vi "about.vi"(7 "httpRequestID":u32) -> ()   [LabVIEW 2011]
doc: "This VI is a state machine that can be ran from a Browser."
uses:
  server/database/Users/User Record.ctl
  <vilib>/wsapi/NI_WebServices.lvlib
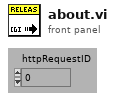
[diagram p1: front panel]
types:
  T1 = typedef "User Record.ctl" = cluster{"ixUser":i32, "sxUsername":string, "sLastName":string, "sFirstName":string, "sEmail":string, "sPassword":string, "tLoginTime":timestamp, "sLoginComputer":string, "fAdministrator":bool, "fRunSequences":bool, "fModifySequences":bool, "fRunScenarios":bool, "fModifyScenarios":bool, "fModifyTemplates":bool, "fModifyUsers":bool, "fModifyStations":bool, "fModifyFields":bool}
  T2 = typedef "Connection Refnum.ctl" = cluster{"Environment Handle":i32, "Connection Handle":i32}
  T3 = typedef "Keyed Array.ctl" = cluster{"keys":string[], "values":string[]}
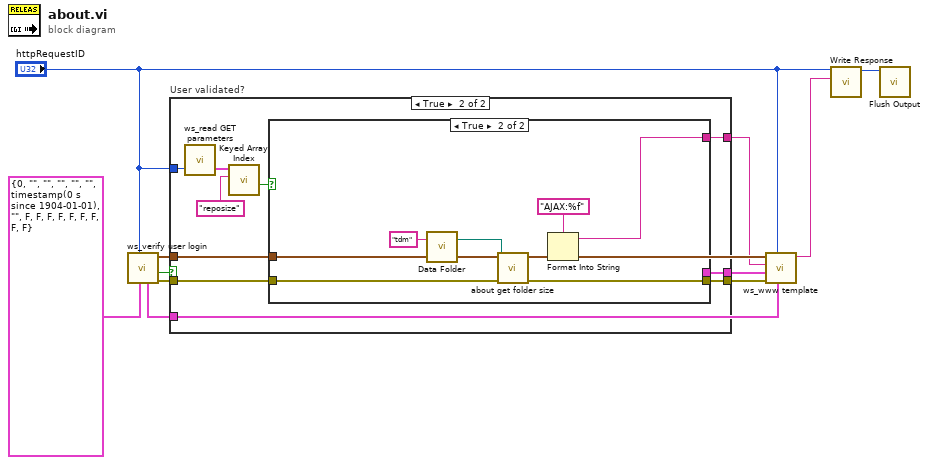
[diagram p0: block diagram]
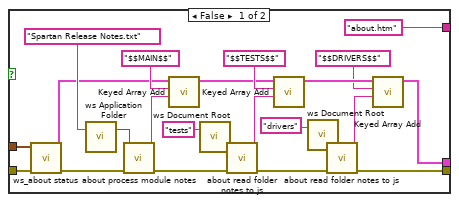
[diagram p3: hidden frame]
diagram:
  n1 = call "ws_verify user login.vi"("Required Permisions"=T1 {"ixUser"=0, "sxUsername"="", "sLastName"="", "sFirstName"="", "sEmail"="", "sPassword"="", "tLoginTime"=timestamp(0 s since 1904-01-01), "sLoginComputer"="", "fAdministrator"=FALSE, "fRunSequences"=FALSE, "fModifySequences"=FALSE, "fRunScenarios"=FALSE, "fModifyScenarios"=FALSE, "fModifyTemplates"=FALSE, "fModifyUsers"=FALSE, "fModifyStations"=FALSE, "fModifyFields"=FALSE} ("User Record"), "httpRequestID"="httpRequestID") -> ("error out"=w9:errorcluster, "User Verified\nand Spartan\nAuthorized?"=w11:bool, "DB Connection Ref"=w6:T2, "User"=w3:T1)  [unwired: 6 in]
  n2 = case "User validated?" shown="True" w11 {
    tunnel: [w12 w18] -> w7
    tunnel: [_ w21] -> w4
    tunnel: [_ w20] -> w5
    tunnel: w3 -> [_ _]
    tunnel: w9 -> [w12 w19]
    tunnel: w6 -> [_ w17]
    tunnel: "httpRequestID" -> [_ w16]
    frame False {
    }
    frame True {
      n3 = call "ws_read GET parameters.vi"("httpRequestID"=w16) -> ("GET query params"=w15:T3)  [unwired: 2 in]
      n4 = call <vilib>:"Keyed Array Index.vi"("key"="reposize", "array in"=w15) -> ("valid key"=w14:bool)  [unwired: 2 in, 3 out]
      n5 = case shown="True" w14 {
        tunnel: ["about.htm" ("Template (\"\")") w50] -> w21
        tunnel: [w41 _] -> w20
        tunnel: w19 -> [w32 w49]
        tunnel: [w31 w45] -> w18
        tunnel: w17 -> [w28 _]
        frame False {
          n6 = call "ws_about status.vi"("error in (no error)"=w32, "Connection Refnum"=w28) -> ("error out"=w35:errorcluster, "keys"=w25:T3)  [unwired: 8 in]
          n7 = call "ws Application Folder.vi"("Relative Path (\"\" - Folder)"="Spartan Release Notes.txt" ("name or relative path")) -> ("Application Folder"=w33:path)  [unwired: 2 in]
          n8 = call "about process module notes.vi"("error in (no error)"=w35, "Notes Path (empty)"=w33) -> ("error out"=w34:errorcluster, "release notes obj"=w29:string)  [unwired: 8 out]
          n9 = call <vilib>:"Keyed Array Add.vi"("value"=w29, "key"="$$MAIN$$" ("Template (\"\")"), "array in"=w25) -> ("array out"=w39:T3)  [unwired: 2 in, 2 out]
          n10 = call "ws Document Root.vi"("Relative Path (\"\" - Folder)"="tests" ("Template (\"\")")) -> ("DocumentRoot Folder"=w37:path)  [unwired: 2 in]
          n11 = call "about read folder notes to js.vi"("error in (no error)"=w34, "Modules Path (empty)"=w37) -> ("error out"=w36:errorcluster, "Module Notes objects"=w27:string)  [unwired: 8 out]
          n12 = call <vilib>:"Keyed Array Add.vi"("value"=w27, "key"="$$TESTS$$" ("Template (\"\")"), "array in"=w39) -> ("array out"=w42:T3)  [unwired: 2 in, 2 out]
          n13 = call "ws Document Root.vi"("Relative Path (\"\" - Folder)"="drivers" ("Template (\"\")")) -> ("DocumentRoot Folder"=w23:path)  [unwired: 2 in]
          n14 = call "about read folder notes to js.vi"("error in (no error)"=w36, "Modules Path (empty)"=w23) -> ("error out"=w31:errorcluster, "Module Notes objects"=w26:string)  [unwired: 8 out]
          n15 = call <vilib>:"Keyed Array Add.vi"("value"=w26, "key"="$$DRIVERS$$" ("Template (\"\")"), "array in"=w42) -> ("array out"=w41:T3)  [unwired: 2 in, 2 out]
        }
        frame True {
          n16 = call "Data Folder.vi"("Relative Path (\"\" - Folder)"="tdm" ("Relative Path (\"\" - Folder)")) -> ("Data Folder"=w48:path)  [unwired: 2 in]
          n17 = call "about get folder size.vi"("error in (no error)"=w49, "Directory Path"=w48) -> ("error out"=w45:errorcluster, "Disk Space Used (MB)"=w46:dbl)  [unwired: 8 in]
          n18 = Format Into String(format string="AJAX:%f" ("Template (\"\")"), w46) -> (resulting string=w50:string)  [unwired: 2 in, 1 out]
        }
      }
    }
  }
  n19 = call "ws_www template.vi"("User"=w3, "httpRequestID"="httpRequestID", "error in (no error)"=w7, "Template Keys (empty)"=w5, "Template (\"\")"=w4, "DB Connection Ref"=w6) -> ("HTTP Template Content"=w2:string)  [unwired: 5 in]
  n20 = call <vilib>:"Write Response.vi"("response string"=w2, "httpRequestID"="httpRequestID") -> ("httpRequestID out"=w8:u32)  [unwired: 8 in, 1 out]
  n21 = call <vilib>:"Flush Output.vi"("httpRequestID"=w8) -> ()  [unwired: 9 in, 2 out]
